vi "Scan Properties.vi"(8 "error in (no error)":errorcluster, 11 "Application":refnum<k7>) -> (0 "error out":errorcluster, 3 "Scan Properties":T1)   [LabVIEW 2020]
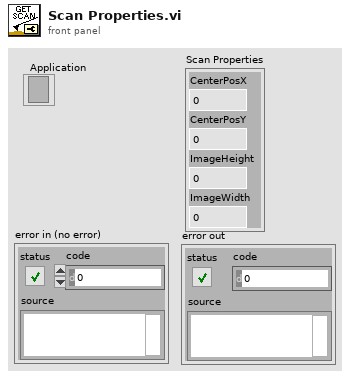
[diagram p1: front panel]
types:
  T1 = cluster{"CenterPosX":dbl, "CenterPosY":dbl, "ImageHeight":dbl, "ImageWidth":dbl}
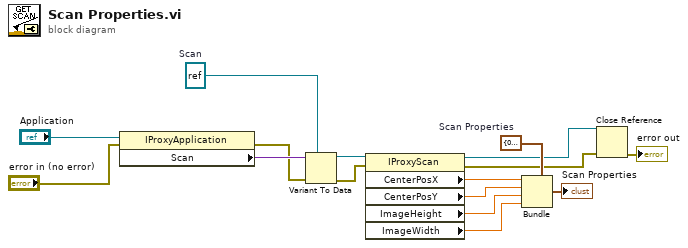
[diagram p0: block diagram]
diagram:
  w8 = T1 {"CenterPosX"=0.0, "CenterPosY"=0.0, "ImageHeight"=0.0, "ImageWidth"=0.0}  # Scan Properties
  w14 = refnum<k7> refnum  # Scan
  n1 = property class="IProxyApplication"(reference="Application", error in="error in (no error)") -> (error out=w3:errorcluster, "Scan"=w15:variant)  [unwired: 1 out]
  n2 = Variant To Data(error in=w3, type=w14, Variant=w15) -> (data=w13:refnum<k7>, error out=w4:errorcluster)
  n3 = property class="IProxyScan"(reference=w13, error in=w4) -> (reference out=w6:refnum<k7>, error out=w5:errorcluster, "CenterPosX"=w12:dbl, "CenterPosY"=w11:dbl, "ImageHeight"=w10:dbl, "ImageWidth"=w9:dbl)
  n4 = Bundle(cluster=w8, "CenterPosX"=w12, "CenterPosY"=w11, "ImageHeight"=w10, "ImageWidth"=w9) -> (→"Scan Properties":T1)
  n5 = Close Reference(reference=w6, error in (no error)=w5) -> (error out=→"error out":errorcluster)
